vi "MC5e Gobal_Variables.vi"() -> ()   [LabVIEW 2020]
uses:
  MC5e Command Q.ctl
  MC5e Data_Parameters.ctl
  MC5e Force.ctl
  MC5e Unit.ctl
  MC5e Unit_Status_List.ctl
  MC5e Squad_Info.ctl
  MC5e Terrain types.ctl
  MC5e Size_Categories.ctl
  Location.ctl
panel:
  in  "Data Parameters":T1
  in  "Command Q":T9={"Command"="Initialize", "Data String"="", "Variant"=variant}
  out "Revision Number":i32
  in  "filename time format":string="%Y%m%d_%H%M%S%3u"
  in  "general timestamp format":string="%m/%d/%Y %I:%M:%S%3u %p"
  in  "Default Public Path":path=path "C:/Users/Public/Documents/National Instruments/BLISS Image Sampler"
  out "Exit":bool
  # "Squads are restricted to one type of soldier (i.e  Archers) and all of the same level.\nIf you want mixed CR or mixed types, use multiple squads."
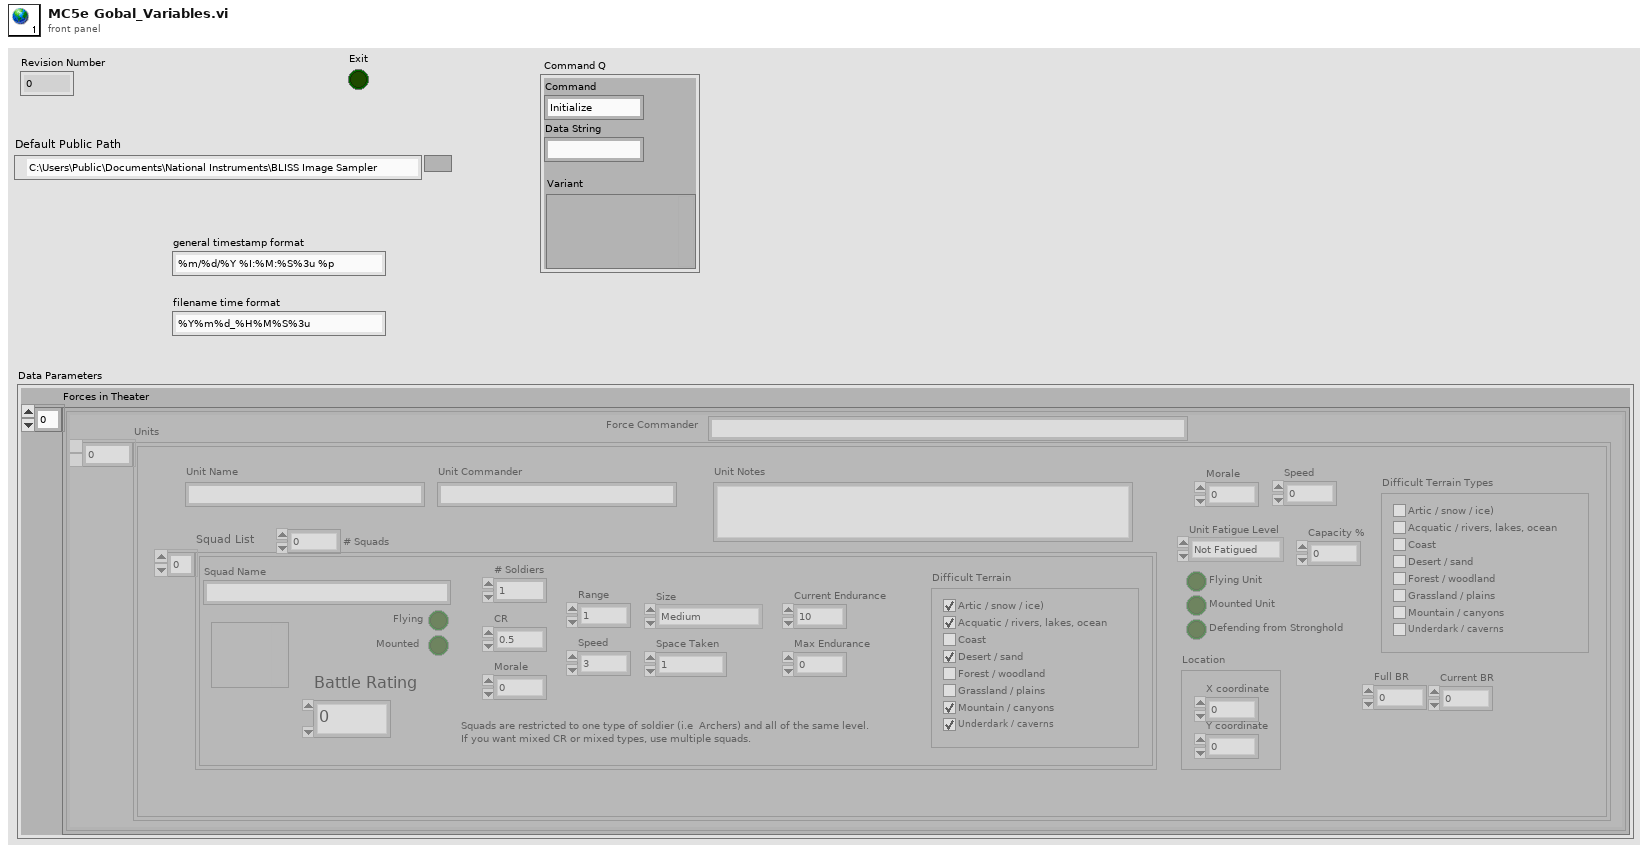
[diagram p1: front panel]
types:
  T1 = typedef "MC5e Data_Parameters.ctl" = cluster{"Forces in Theater":T2[]}
  T2 = typedef "MC5e Force.ctl" = cluster{"Force Commander":string, "Units":T3[]}
  T3 = typedef "MC5e Unit.ctl" = cluster{"Squad List":T4, "Unit Fatigue Level":enum16{"Not Fatigued", "Fatigued", "Seriously Fatigued"}, "Flying Unit":bool, "Mounted Unit":bool, "Difficult Terrain Types":T6, "Full BR":dbl, "Defending from Stronghold":bool, "Speed":dbl, "Capacity %":dbl, "Morale":dbl, "Current BR":dbl, "Location":T8, "Unit Name":string, "Unit Commander":string, "Unit Notes":string, "# Squads":dbl}
  T4 = typedef "MC5e Unit_Status_List.ctl" = T5[]
  T5 = typedef "MC5e Squad_Info.ctl" = cluster{"Squad Name":string, "# Soldiers":dbl, "Battle Rating":dbl, "Flying":bool, "Mounted":bool, "Speed":dbl, "Range":dbl, "Morale":dbl, "Token Image":variant, "Max Endurance":dbl, "Current Endurance":dbl, "Difficult Terrain":T6, "Size":T7, "Space Taken":dbl, "CR":dbl}
  T6 = typedef "MC5e Terrain types.ctl" = cluster{"Artic / snow / ice)":bool, "Coast":bool, "Desert / sand":bool, "Forest / woodland":bool, "Grassland / plains":bool, "Mountain / canyons":bool, "Underdark / caverns":bool, "Acquatic / rivers, lakes, ocean":bool}
  T7 = typedef "MC5e Size_Categories.ctl" = enum16{"Tiny", "Small", "Medium", "Large", "Huge", "Gargantuan"}
  T8 = typedef "Location.ctl" = cluster{"X coordinate":dbl, "Y coordinate":dbl}
  T9 = typedef "MC5e Command Q.ctl" = cluster{"Command":string, "Data String":string, "Variant":variant}
diagram:
